vi "Beam-Breaker-Out.vi"() -> (2 "PASSED-OUT?":bool)   [LabVIEW 2019]
uses:
  Robot Global Data.vi
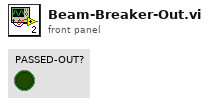
[diagram p1: front panel]
types:
  T1 = typedef "WPI_DigitalOutputDevRef.ctl" = cluster{"DIO Channel":T2, "DevStatus":errorcluster}
  T2 = typedef "FPGA_DIOChannel.ctl" = enum8{"DIO 0", "DIO 1", "DIO 2", "DIO 3", "DIO 4", "DIO 5", "DIO 6", "DIO 7", "DIO 8", "DIO 9", "DIO MXP 0", "DIO MXP 1", "DIO MXP 2", "DIO MXP 3", "DIO MXP 4", "DIO MXP 5", "DIO MXP 6", "DIO MXP 7", "DIO MXP 8", "DIO MXP 9", "DIO MXP 10", "DIO MXP 11", "DIO MXP 12", "DIO MXP 13", "DIO MXP 14", "DIO MXP 15", "SPI Port CS1", "SPI Port CS2", "SPI Port CS3", "SPI Port MISO", "SPI Port MOSI", "Invalid"}
  T3 = typedef "WPI_DigitalInputDevRef.ctl" = cluster{"DevStatus":errorcluster, "DIO Channel":T2}
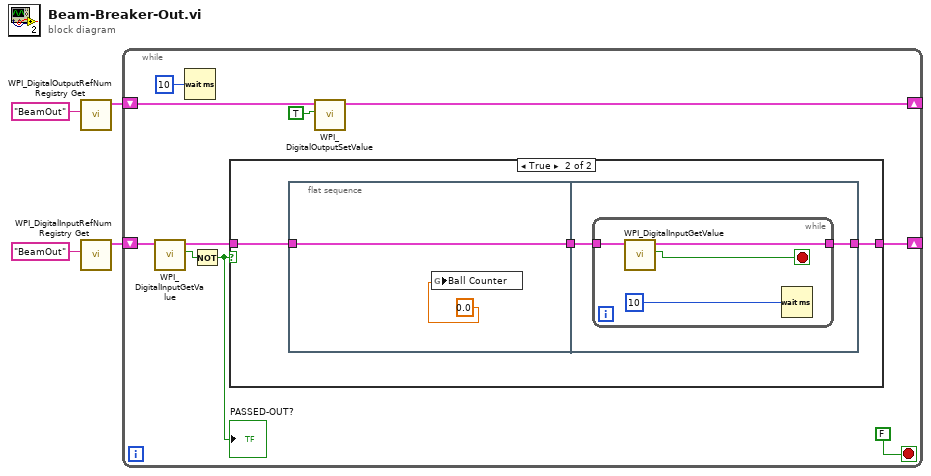
[diagram p0: block diagram]
diagram:
  n1 = call <vilib>:"WPI_DigitalOutputRefNum Registry Get.vi"("refnum name"="BeamOut") -> ("DigitalOutputDevRef"=w2:T1)  [unwired: 9 in, 1 out]
  n2 = call <vilib>:"WPI_DigitalInputRefNum Registry Get.vi"("refnum name"="BeamOut") -> ("DigitalInputDevRef"=w3:T3)  [unwired: 9 in, 1 out]
  n3 = while {
    shift-right: [w11] -> _
    shift-left: w3 -> [w14]
    shift-right: [w9] -> _
    shift-left: w2 -> [w10]
    stop <- FALSE stop-if-true
    n4 = call <vilib>:"WPI_DigitalInputGetValue.vi"("DigitalInputDevRef"=w14) -> ("Value"=w6:bool, "DigitalInputDevRef"=w12:T3)  [unwired: 8 in, 1 out]
    n5 = Wait (ms)(milliseconds to wait=u32 10 ("millisecond timer value")) -> ()  [unwired: 1 out]
    n6 = Not(x=w6) -> (.not. x?=w5:bool)
    "PASSED-OUT?" <- w5
    n7 = case shown="True" w5 {
      tunnel: w12 -> [w15 w17]
      tunnel: [w15 w18] -> w11
      frame False {
      }
      frame True {
        n8 = flat-sequence {
          tunnel: w17 -> [w20]
          tunnel: [w20] -> w16
          tunnel: [w22] -> w18
          tunnel: w16 -> [w21]
          frame #0 {
            n9 = global write "Robot Global Data.vi" "Ball Counter"(0.0 ("Ball Counter")) -> ()
          }
          frame #1 {
            n10 = while {
              tunnel: w21 -> [w25]
              tunnel: [w24] -> w22
              stop <- w23 stop-if-true
              n11 = call <vilib>:"WPI_DigitalInputGetValue.vi"("DigitalInputDevRef"=w25) -> ("Value"=w23:bool, "DigitalInputDevRef"=w24:T3)  [unwired: 8 in, 1 out]
              n12 = Wait (ms)(milliseconds to wait=u32 10) -> ()  [unwired: 1 out]
            }
          }
        }
      }
    }
    n13 = call <vilib>:"WPI_DigitalOutputSetValue.vi"("Value"=TRUE, "DigitalOutputDevRef"=w10) -> ("DigitalOutputDevRef"=w9:T1)  [unwired: 8 in, 1 out]
  }
